vi "XNET Read (Frame CAN RT).vi"(0 "session in":refnum<k21>, 5 "data in":T1[](array[typedef]) {"payload" format="%x"; "timestamp" format="%<%.7X\n%x>T"; "type" items=["CAN Data"=0, "CAN Remote"=1, "CAN Bus Error"=2, "CAN 2.0 Data"=8, "CAN FD Data"=16, "CAN FD+BRS Data"=24, "J1939 Data"=192, "Delay"=224, "Log Trigger"=225, "Start Trigger"=226]; "identifier" format="%x"}, 7 "number to read (-1)":i32=-1, 9 "timeout (0)":dbl format="%.2g", 11 "error in (no error)":errorcluster, 12 "unused payloads in":cluster{"payload":u8[]}[](array[cluster])) -> (4 "session out":refnum<k21>, 6 "data":T1[](array[typedef]) {"payload" format="%x"; "timestamp" format="%<%.7X\n%x>T"; "type" items=["CAN Data"=0, "CAN Remote"=1, "CAN Bus Error"=2, "CAN 2.0 Data"=8, "CAN FD Data"=16, "CAN FD+BRS Data"=24, "J1939 Data"=192, "Delay"=224, "Log Trigger"=225, "Start Trigger"=226]; "identifier" format="%x"}, 14 "unused payloads":cluster{"payload":u8[]}[](array[cluster]), 15 "error out":errorcluster)   [LabVIEW 2018]
doc: "Reads data from a session as an array of CAN frames. The session must use a CAN interface and a mode of Frame Input Stream, Frame Input Queued, or Frame Input Single-Point.\n\nThis Real-Time (RT) version of XNET Read (Frame CAN) can be used to workaround performance problems in LabVIEW related to the CAN frame data type (array of cluster with array).\n\nIn LabVIEW versions 8.6 and higher, the performance issues are limited to jitter in high-priority loops on LabVIEW Real-Time (RT). To use this VI, wire the \"data\" and \"unused payloads\"\ninput/output to a shift register in all loops that contain the Read. The initial value of each can use the default constant (empty array)."
uses:
  XNET Frame CAN.ctl
  XNET Frame Type CAN.ctl
  nixlvapi.dll
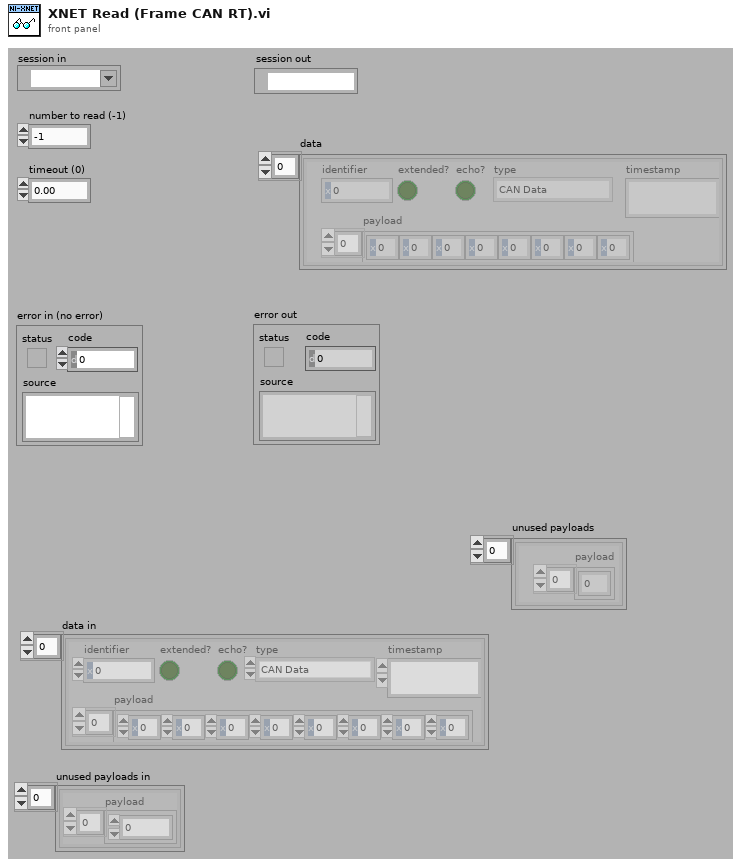
[diagram p1: front panel]
types:
  T1 = typedef "XNET Frame CAN.ctl" = cluster{"timestamp":timestamp, "payload":u8[], "identifier":u32, "type":T2, "extended?":bool, "echo?":bool}
  T2 = typedef "XNET Frame Type CAN.ctl" = u8
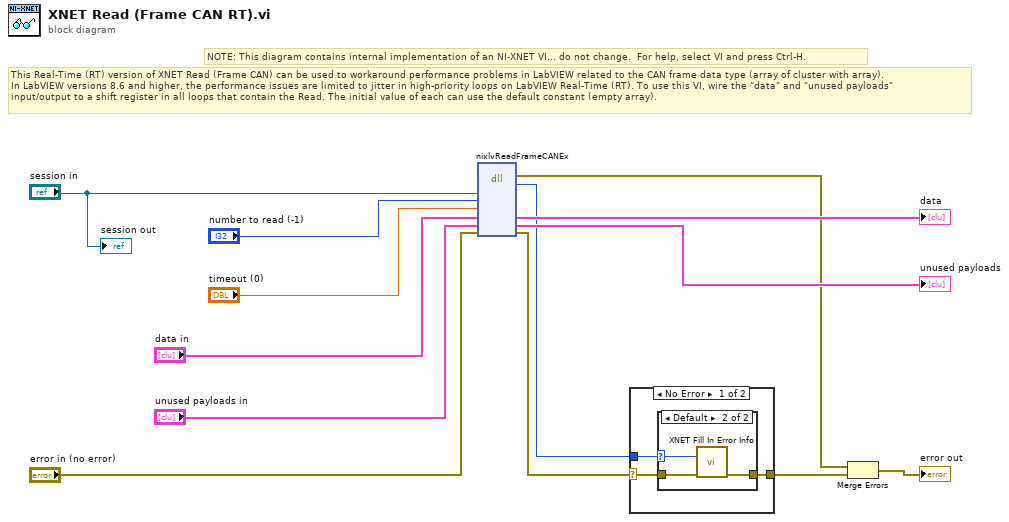
[diagram p0: block diagram]
diagram:
  # "This Real-Time (RT) version of XNET Read (Frame CAN) can be used to workaround performance problems in LabVIEW related to the CAN frame data type (array of cluster with array).\nIn LabVIEW versions 8.6 and higher, the performance issues are limited to jitter in high-priority loops on LabVIEW Real-Time (RT). To use this VI, wire the \"data\" and \"unused payloads\"\ninput/output to a shift register in all loops that contain the Read. The initial value of each can use the default constant (empty array)."
  # "NOTE: This diagram contains internal implementation of an NI-XNET VI... do not change.  For help, select VI and press Ctrl-H."
  n1 = dll-call lib="nixlvapi.*" fn="nixlvReadFrameCANEx" label="Call Library"("sessionRef"="session in", "numberToRead"="number to read (-1)", "timeout"="timeout (0)", "lvData"="data in", "unusedPayloads"="unused payloads in", "errorInOut"="error in (no error)") -> (error out=w1:errorcluster, "return type"=w4:i32, "lvData"=→"data":T1[], "unusedPayloads"=→"unused payloads":cluster{"payload":u8[]}[], "errorInOut"=w3:errorcluster)  [unwired: 5 in, 2 out]
  n2 = case shown="No Error" w3 {
    selector: w3 -> [w14 w21]
    tunnel: [w16 w21] -> w13
    tunnel: w4 -> [w15 _]
    frame No Error {
      n3 = case shown="Default" w15 {
        selector: w15 -> [_ w18]
        tunnel: w14 -> [w17 w19]
        tunnel: [w17 w20] -> w16
        frame 0 {
        }
        frame Default {
          n4 = call "XNET Fill In Error Info.vi"("status code"=w18, "error in"=w19) -> ("error out"=w20:errorcluster)  [unwired: 13 out]
        }
      }
    }
    frame Error {
    }
  }
  n5 = Merge Errors(w1, w13) -> (→"error out":errorcluster)
  "session out" <- "session in"
